vi "PCO_GetWhiteBalance.vi"(0 "ph":u64, 1 "mode":i32, 2 "width":i32, 3 "height":i32, 4 "gb12":u16[][](array[numeric])=array1x4097[4097 elements], 5 "x_min":i32, 6 "y_min":i32, 7 "error in (no error)":errorcluster {"code" format="%x"}, 8 "x_max":i32, 9 "y_max":i32) -> (20 "ph out":u64, 21 "ErrorMessage":i32 format="%x", 22 "color_temp":i32, 23 "tint":i32, 27 "error out":errorcluster {"code" format="%x"})   [LabVIEW 2019, in "Convert.lvlib"]
doc: "int PCOCONVERT_API PCO_GetWhiteBalance(HANDLE ph, int *color_temp, int *tint, int mode, int width, int height, word *gb12, int x_min, int y_min, int x_max, int y_max);"
uses:
  Convert.lvlib
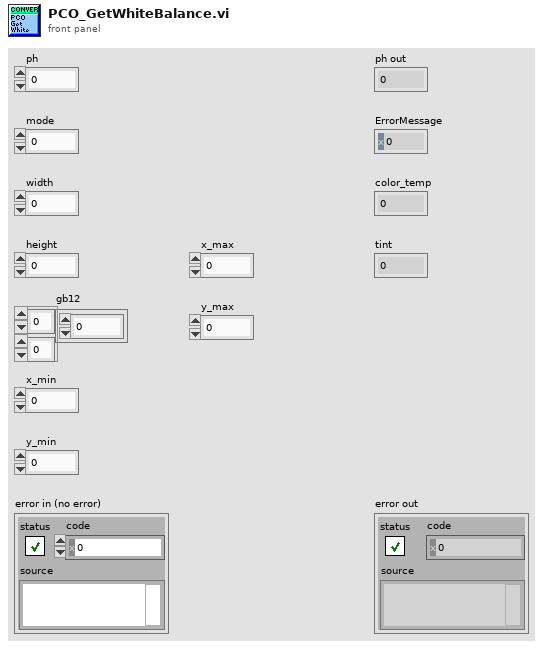
[diagram p1: front panel]
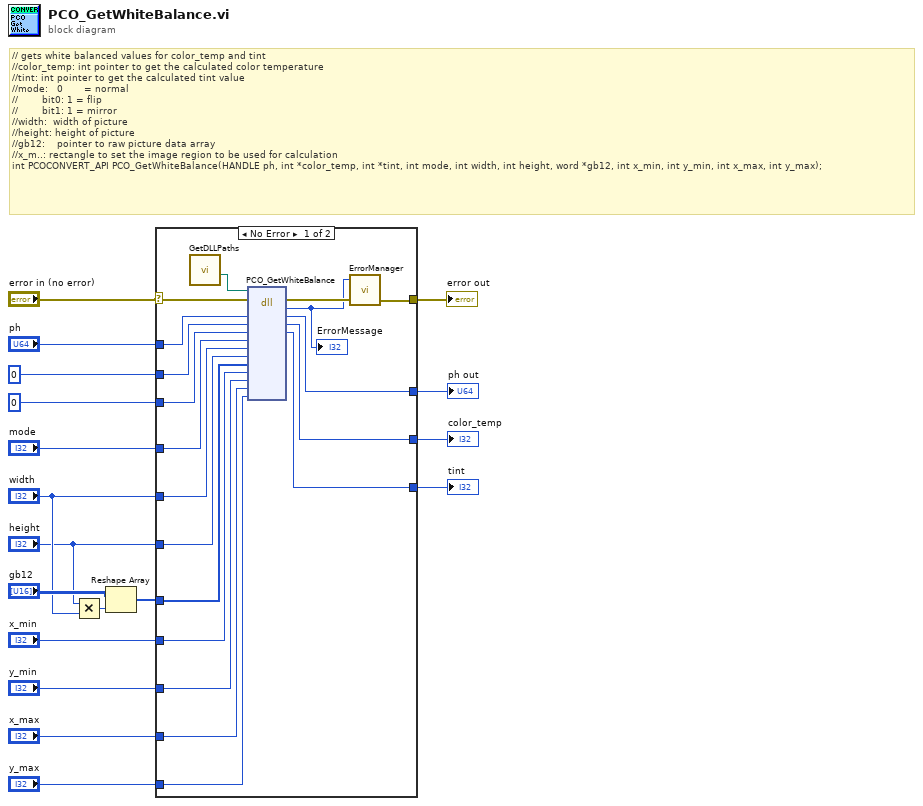
[diagram p0: block diagram]
diagram:
  # "// gets white balanced values for color_temp and tint\n//color_temp: int pointer to get the calculated color temperature\n//tint: int pointer to get the calculated tint value\n//mode:   0       = normal\n//        bit0: 1 = flip\n//        bit1: 1 = mirror  \n//width:  width of picture\n//height: height of picture\n//gb12:    pointer to raw picture data array\n//x_m..: rectangle to set the image region to be used for calculation\nint PCOCONVERT_API PCO_GetWhiteBalance(HANDLE ph, int *color_temp, int *tint, int mode, int width, int height, word *gb12, int x_min, int y_min, int x_max, int y_max);"
  n1 = Multiply(x="height", y="width") -> (x*y=w5:i32)
  n2 = Reshape Array("gb12", w5) -> (w1:u16[])
  n3 = case shown="No Error" "error in (no error)" {
    selector: "error in (no error)" -> [w21 w41]
    tunnel: "ph" -> [w37 w40]
    tunnel: [w36 w40] -> w17
    tunnel: 0 ("color_temp") -> [w35 w39]
    tunnel: [w34 w39] -> w15
    tunnel: 0 ("tint") -> [w33 w38]
    tunnel: [w32 w38] -> w13
    tunnel: "mode" -> [w31 _]
    tunnel: "width" -> [w30 _]
    tunnel: "height" -> [w29 _]
    tunnel: w1 -> [w28 _]
    tunnel: "x_min" -> [w27 _]
    tunnel: "y_min" -> [w26 _]
    tunnel: "x_max" -> [w25 _]
    tunnel: "y_max" -> [w24 _]
    tunnel: [w22 w41] -> w7
    frame No Error {
      n4 = call "GetDLLPaths.vi"() -> ("PCO_Conv_Path"=w19:path)  [unwired: 8 in, 3 out]
      n5 = dll-call lib="?" fn="PCO_GetWhiteBalance"(path in=w19, error in=w21, "ph"=w37, "color_temp"=w35, "tint"=w33, "mode"=w31, "width"=w30, "height"=w29, "gb12"=w28, "x_min"=w27, "y_min"=w26, "x_max"=w25, "y_max"=w24) -> (error out=w23:errorcluster, "return type"=w20:i32, "ph"=w36:u64, "color_temp"=w34:i32, "tint"=w32:i32)  [unwired: 9 in, 1 out]
      "ErrorMessage" <- w20
      n6 = call "ErrorManager.vi"("error in (no error)"=w23, "error code"=w20) -> ("error out"=w22:errorcluster)  [unwired: 2 in, 1 out]
    }
    frame Error {
    }
  }
  "ph out" <- w17
  "color_temp" <- w15
  "tint" <- w13
  "error out" <- w7
